vi "Scale Channel (Scalar).vi"(9 "Value":dbl, 10 "Scaling Params":dbl[](array[numeric]), 11 "Scaling Type":T1) -> (1 "Scaled Value":dbl)   [LabVIEW 2020, in "VolatusData.lvlib" / "Scaling.lvclass"]
uses:
  Scaling.lvclass
  VolatusConfig/Scale Type.ctl
  Polynomial Remove Trailing Zeros.vi
  Scaling.lvclass/Scaling.ctl
  VolatusConfig/VolatusConfig.lvlib
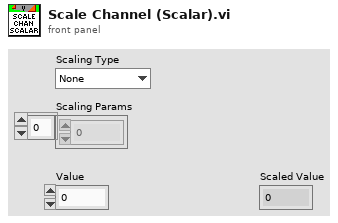
[diagram p1: front panel]
types:
  T1 = typedef "VolatusConfig.lvlib/Scale Type.ctl" = enum16{"None", "Sensor", "Polynomial", "Threshold", "Invert Bool"}
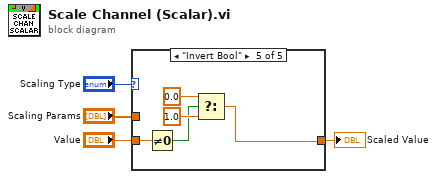
[diagram p0: block diagram]
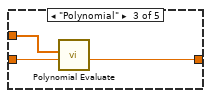
[diagram p4: hidden frame]
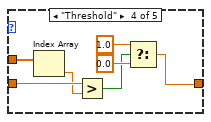
[diagram p5: hidden frame]
diagram:
  n1 = case shown="\"Invert Bool\"" "Scaling Type" {
    tunnel: "Scaling Params" -> [_ _ w9 w16 _]
    tunnel: "Value" -> [w5 w6 w8 w15 w21]
    tunnel: [w5 w6 w7 w10 w17] -> w1
    frame "None" {
    }
    frame "Sensor" {
      # "#ERROR?\nSensor should be converted to another type."
    }
    frame "Polynomial" {
      n2 = call "Polynomial Evaluate.vi"("Data"=w8, "Coefficients"=w9) -> ("Results"=w7:dbl)  [unwired: 9 in]
    }
    frame "Threshold" {
      n3 = Index Array(array=w16) -> (element=w14:dbl)  [unwired: 1 in]
      n4 = Greater?(x=w15, y=w14) -> (0:w11:bool)
      n5 = Select(t=1.0, s=w11, f=0.0) -> (s? t:f=w10:dbl)
    }
    frame "Invert Bool" {
      n6 = Not Equal To 0?(x=w21) -> (x != 0?=w18:bool)
      n7 = Select(t=0.0, s=w18, f=1.0) -> (s? t:f=w17:dbl)
    }
  }
  "Scaled Value" <- w1
